vi "logging_info_write.vi"(7 "Add call chain offset\n(No call chain)":i32=-1, 8 "error in":errorcluster caption="error in (no error)", 10 "String to write":string, 11 "VISA resource name":refnum<visa-resource-name>) -> (0 "error out":errorcluster, 3 "VISA resource name out":refnum<visa-resource-name>)   [LabVIEW 2020, in "Rohde&Schwarz RTx Oscilloscopes.lvlib" / "rsidr_core.lvlib"]
uses:
  rsidr_core.lvlib
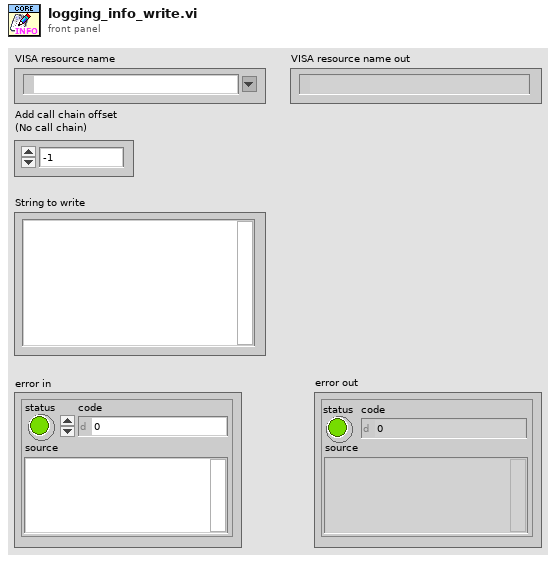
[diagram p1: front panel]
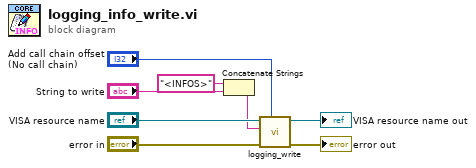
[diagram p0: block diagram]
diagram:
  n1 = Concatenate Strings("<INFOS>" ("string"), "String to write") -> (w2:string)
  n2 = call "logging_write.vi"("Add call chain offset\n(No call chain)"="Add call chain offset\n(No call chain)", "error in"="error in", "String to write"=w2, "VISA resource name"="VISA resource name") -> ("error out"=→"error out":errorcluster, "VISA resource name out"=→"VISA resource name out":refnum<visa-resource-name>)  [unwired: 6 in]
